vi "FPGA Main.vi"   [LabVIEW 2019]
uses:
  <vilib>/rvi/Emulation/niFpgaGetClockAttributes.vi
  <vilib>/rvi/Emulation/niFpgaSctlEmulationGetInTimedLoop.vi
  <vilib>/rvi/Emulation/niFpgaEmulationReportErrorSimple.vi
  <vilib>/rvi/eio/common/nirviEmuTemplateMethod_errors.vi
  <vilib>/rvi/Emulation/niFpgaCriticalErrorInLSC.vi
  <vilib>/eio/EIONode/EIONode.xnode
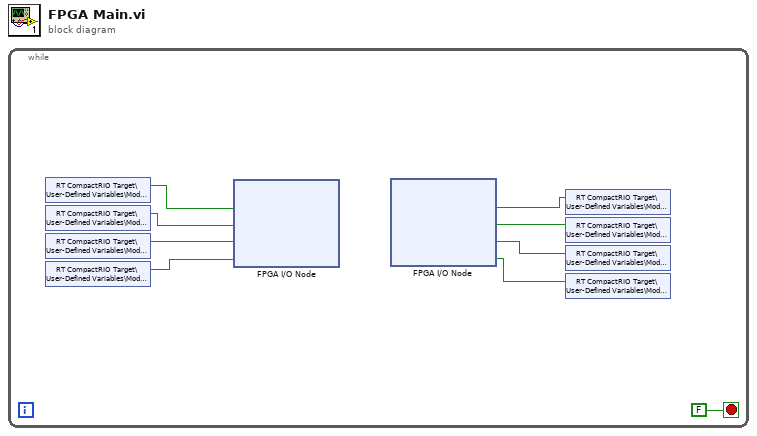
[diagram p0: block diagram]
diagram:
  n1 = while {
    stop <- FALSE stop-if-true
    n2 = shared-variable "RT CompactRIO Target\\User-Defined Variables\\Mod7 DIO0"() -> (w2:bool)  [unwired: 1 in, 1 out]
    n3 = shared-variable "RT CompactRIO Target\\User-Defined Variables\\Mod7 DIO1"() -> (w3:bool)  [unwired: 1 in, 1 out]
    n4 = shared-variable "RT CompactRIO Target\\User-Defined Variables\\Mod7 DIO2"() -> (w4:bool)  [unwired: 1 in, 1 out]
    n5 = shared-variable "RT CompactRIO Target\\User-Defined Variables\\Mod7 DIO3"() -> (w5:bool)  [unwired: 1 in, 1 out]
    n6 = xnode "FPGA I/O Node"("Mod7/DIO0"=w2, "Mod7/DIO1"=w3, "Mod7/DIO2"=w4, "Mod7/DIO3"=w5) -> ()  [unwired: 4 in, 4 out]
    n7 = xnode "FPGA I/O Node"() -> ("Mod6/DIO0"=w9:bool, "Mod6/DIO1"=w8:bool, "Mod6/DIO2"=w7:bool, "Mod6/DIO3"=w6:bool)  [unwired: 4 in, 4 out]
    n8 = shared-variable "RT CompactRIO Target\\User-Defined Variables\\Mod6 DIO0"(w9) -> ()  [unwired: 1 in, 1 out]
    n9 = shared-variable "RT CompactRIO Target\\User-Defined Variables\\Mod6 DIO1"(w8) -> ()  [unwired: 1 in, 1 out]
    n10 = shared-variable "RT CompactRIO Target\\User-Defined Variables\\Mod6 DIO2"(w7) -> ()  [unwired: 1 in, 1 out]
    n11 = shared-variable "RT CompactRIO Target\\User-Defined Variables\\Mod6 DIO3"(w6) -> ()  [unwired: 1 in, 1 out]
  }
